vi "Compute Offset and round-trip time.vi"() -> ()   [LabVIEW 2013]
panel:
  out "t0+t3":dbl format="%.6f"
  out "t1+t2":dbl format="%.6f"
  out "Round-Trip (s)":dbl
  out "Offset (s)":dbl
  out "t 3":dbl format="%.6f"
  out "t 2":dbl format="%.6f"
  out "t 1":dbl format="%.6f"
  out "t 0":dbl format="%.6f"
  in  "Server Time (Receive TimeStamp)":timestamp=timestamp(3518362050.498921 s since 1904-01-01) format="%<%.6X\n%x>T"
  in  "current time":timestamp=timestamp(3518362050.4889207 s since 1904-01-01) format="%<%.6X\n%x>T"
  in  "Local Time (Destination TimeStamp)":timestamp=timestamp(3518362050.509195 s since 1904-01-01) format="%<%.6X\n%x>T"
  in  "Server Time (Transmit TimeStamp)":timestamp=timestamp(3518362050.4989305 s since 1904-01-01) format="%<%.6X\n%x>T"
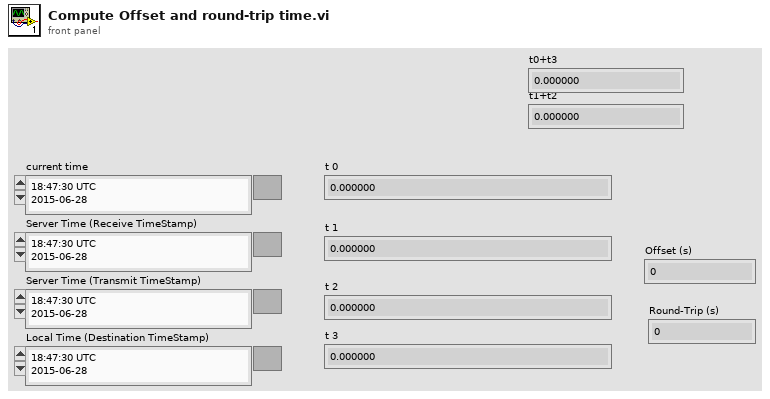
[diagram p1: front panel]
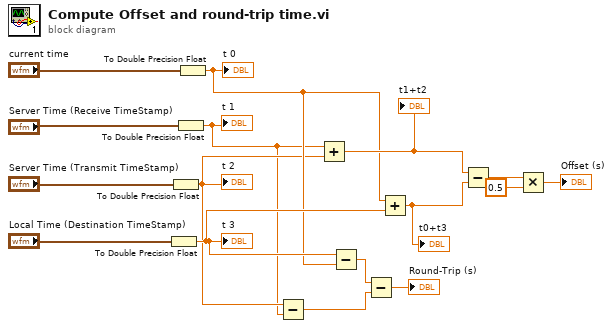
[diagram p0: block diagram]
diagram:
  n1 = To Double Precision Float(number="Local Time (Destination TimeStamp)") -> (double precision float=w8:dbl)
  "t 3" <- w8
  n2 = To Double Precision Float(number="Server Time (Transmit TimeStamp)") -> (double precision float=w6:dbl)
  "t 2" <- w6
  n3 = To Double Precision Float(number="Server Time (Receive TimeStamp)") -> (double precision float=w5:dbl)
  "t 1" <- w5
  n4 = To Double Precision Float(number="current time") -> (double precision float=w7:dbl)
  "t 0" <- w7
  n5 = Subtract(x=w6, y=w5) -> (x-y=w3:dbl)
  n6 = Add(x=w5, y=w6) -> (x+y=w12:dbl)
  "t1+t2" <- w12
  n7 = Subtract(x=w8, y=w7) -> (x-y=w4:dbl)
  n8 = Subtract(x=w4, y=w3) -> (x-y=→"Round-Trip (s)":dbl)
  n9 = Add(x=w7, y=w8) -> (x+y=w1:dbl)
  "t0+t3" <- w1
  n10 = Subtract(x=w12, y=w1) -> (x-y=w11:dbl)
  n11 = Multiply(x=w11, y=0.5) -> (x*y=→"Offset (s)":dbl)
